vi "Encode Tags.vi"(9 "Echo":bool, 10 "Extended ID":bool, 11 "ISO FD Type":T1) -> (3 "Tags":u8)   [LabVIEW 2021, in "CAN_Logic.lvclass"]
uses:
  CAN_Logic.lvclass
  typedef/ISO FD Frame Type.ctl
  CAN_Logic.lvclass/CAN_Logic.ctl
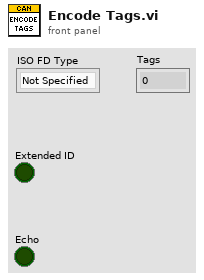
[diagram p1: front panel]
types:
  T1 = typedef "CAN_Logic.lvclass/ISO FD Frame Type.ctl" = enum16{"Not Specified", "CAN 2.0", "FD", "FD+BRS"}
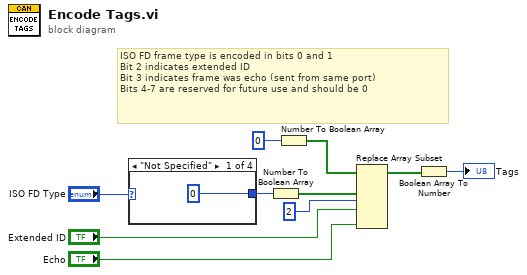
[diagram p0: block diagram]
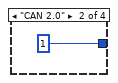
[diagram p2: hidden frame]
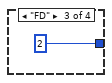
[diagram p3: hidden frame]
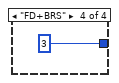
[diagram p4: hidden frame]
diagram:
  # "ISO FD frame type is encoded in bits 0 and 1\nBit 2 indicates extended ID\nBit 3 indicates frame was echo (sent from same port)\nBits 4-7 are reserved for future use and should be 0"
  n1 = case shown="\"Not Specified\"" "ISO FD Type" {
    tunnel: [u8 0 u8 1 u8 2 u8 3] -> w9
    frame "Not Specified" {
    }
    frame "CAN 2.0" {
    }
    frame "FD" {
    }
    frame "FD+BRS" {
    }
  }
  n2 = Number To Boolean Array(number=w9) -> (Boolean array=w6:bool[])
  n3 = Number To Boolean Array(number=u8 0) -> (Boolean array=w4:bool[])
  n4 = Replace Array Subset(array=w4, new element #1=w6, new element #2="Extended ID", index #2=2 ("index"), new element #3="Echo") -> (w2:bool[])  [unwired: 2 in]
  n5 = Boolean Array To Number(Boolean array=w2) -> (number=→"Tags":u8)
